vi "[SubVI]Hip Angle Measurement.vi"(10 "Left Theta":i32, 11 "Right Theta":i32) -> (1 "Left Theta":dbl, 2 "Right Theta":dbl, 3 "Hip Angle Measurement":cluster{dbl, dbl})   [LabVIEW 2017]
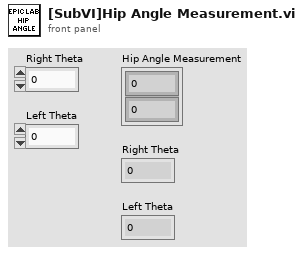
[diagram p1: front panel]
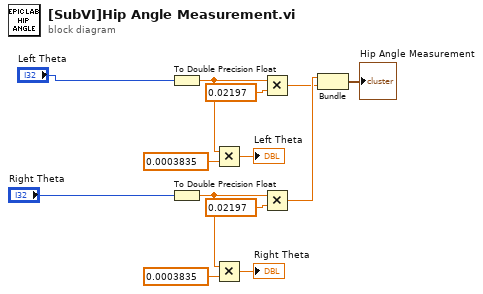
[diagram p0: block diagram]
diagram:
  n1 = To Double Precision Float(number="Left Theta") -> (double precision float=w5:dbl)
  n2 = To Double Precision Float(number="Right Theta") -> (double precision float=w8:dbl)
  n3 = Multiply(x=w5, y=0.0003835) -> (x*y=→"Left Theta":dbl)
  n4 = Multiply(x=w8, y=0.0003835) -> (x*y=→"Right Theta":dbl)
  n5 = Multiply(x=w5, y=0.02197) -> (x*y=w3:dbl)
  n6 = Multiply(x=w8, y=0.02197) -> (x*y=w4:dbl)
  n7 = Bundle(w4, w3) -> (→"Hip Angle Measurement":cluster{dbl, dbl})  [unwired: 1 in]
